vi "word.random_select.vi"(11 "dictonary":string[](array[string])) -> (3 "solution":string)   [LabVIEW 2020, in "Worder.lvclass"]
uses:
  Worder.lvclass
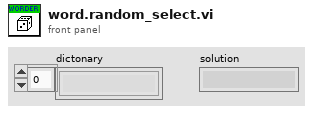
[diagram p1: front panel]
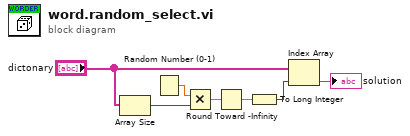
[diagram p0: block diagram]
diagram:
  n1 = Array Size(array="dictonary") -> (size(s)=w1:i32)
  n2 = Random Number (0-1)() -> (number: 0 to 1=w2:dbl)
  n3 = Multiply(x=w2, y=w1) -> (x*y=w3:dbl)
  n4 = Round Toward -Infinity(1:w3) -> (0:w4:dbl)
  n5 = To Long Integer(number=w4) -> (32bit integer=w5:i32)
  n6 = Index Array(array="dictonary", index=w5) -> (element=→"solution":string)
